vi "Simple.vi"() -> ()   [LabVIEW 2018]
uses:
  Spels.AutomationTools.RemoteFunctionalControlService.dll
panel:
  in  "stop":bool
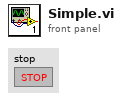
[diagram p1: front panel]
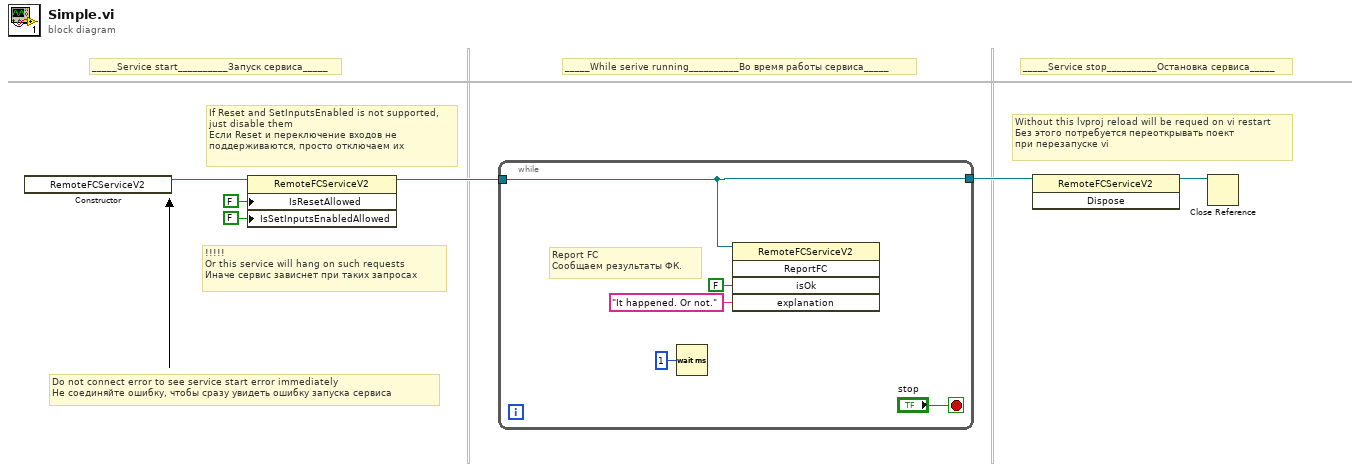
[diagram p0: block diagram]
diagram:
  # "Do not connect error to see service start error immediately\nНе соединяйте ошибку, чтобы сразу увидеть ошибку запуска сервиса"
  # "Without this lvproj reload will be requed on vi restart\nБез этого потребуется переоткрывать поект \nпри перезапуске vi"
  # "_____Service stop__________Остановка сервиса_____"
  # "_____While serive running__________Во время работы сервиса_____"
  # "_____Service start__________Запуск сервиса_____"
  # "!!!!!\nOr this service will hang on such requests\nИначе сервис зависнет при таких запросах"
  # "If Reset and SetInputsEnabled is not supported,\njust disable them\nЕсли Reset и переключение входов не \nподдерживаются, просто отключаем их"
  n1 = constructor class="RemoteFCServiceV2"() -> (reference out=w6:refnum<k24>)  [unwired: 3 in, 2 out]
  n2 = property class="RemoteFCServiceV2"(reference=w6, "IsResetAllowed"=FALSE, "IsSetInputsEnabledAllowed"=FALSE) -> (reference out=w3:refnum<k24>)  [unwired: 1 in, 1 out]
  n3 = while {
    tunnel: [w11] -> w2
    tunnel: w3 -> [w11]
    stop <- "stop" stop-if-true
    # "Report FC\nСообщаем результаты ФК."
    n4 = Wait (ms)(milliseconds to wait=u32 1) -> ()  [unwired: 1 out]
    n5 = invoke class="RemoteFCServiceV2" method="ReportFC"(reference=w11, "isOk"=FALSE, "explanation"="It happened. Or not.") -> ()  [unwired: 2 in, 5 out]
  }
  n6 = invoke class="RemoteFCServiceV2" method="Dispose"(reference=w2) -> (reference out=w1:refnum<k24>)  [unwired: 2 in, 2 out]
  n7 = Close Reference(reference=w1) -> ()  [unwired: 1 in, 1 out]
